vi "Get Buffers.vi"(11 "Transfer in":refnum<class "Transfer.lvclass">) -> (2 "Buffers":refnum<class "Buffers.lvclass">, 3 "Transfer out":refnum<class "Transfer.lvclass">)   [LabVIEW 2021, in "DSF Core.lvlib" / "Transfer.lvclass"]
uses:
  Transfer.lvclass
  Buffers/Buffers.lvclass
  Transfer.lvclass/Transfer.ctl
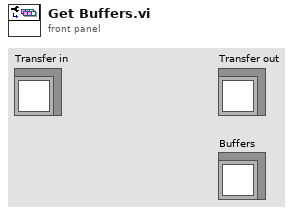
[diagram p1: front panel]
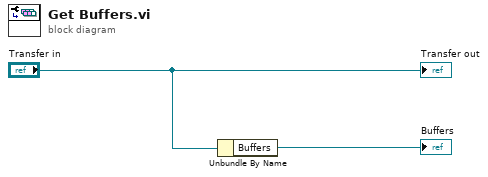
[diagram p0: block diagram]
diagram:
  n1 = Unbundle By Name("Transfer in") -> ("Buffers"=→"Buffers":refnum<class "Buffers.lvclass">)
  "Transfer out" <- "Transfer in"
